vi "log analysis_gps.vi"() -> ()   [LabVIEW 2019] (continued)
-1.127697\t1.583662\t-32.920876\t0.305000\t0.018000\n\t\n15:22:00.9\tlog_raw\tgps_raw\t\tsystem status\tnormal 2 28.100000 0 0\trobot status\t261.941278\t86.398374\t9.062300\t-1.078955\t1.573300\t-32.941024\t0.301000\t0.007000\n\t\n15:22:01.4\tlog_raw\tgps_raw\t\tsystem status\tnormal 2 28.100000 0 0\trobot status\t262.053513\t86.309329\t9.068200\t-0.868450\t1.546924\t-32.927997\t0.298000\t0.007000\n\t\n15:22:02.0\tlog_raw\tgps_raw\t\tsystem status\tnormal 2 28.100000 0 0\trobot status\t262.166872\t86.221531\t9.074900\t-0.908194\t1.762279\t-32.906753\t0.245000\t0.087000\n\t\n15:22:02.4\tlog_raw\tgps_raw\t\tsystem status\tnormal 2 28.100000 0 0\trobot status\t262.277689\t86.134631\t9.082500\t-0.875214\t1.923337\t-32.852666\t0.299000\t0.013000\n\t\n15:22:02.9\tlog_raw\tgps_raw\t\tsystem status\tnormal 2 28.100000 0 0\trobot status\t262.391399\t86.045063\t9.089000\t-0.783137\t1.975369\t-32.776874\t0.269000\t0.061000\n\t\n15:22:03.5\tlog_raw\tgps_raw\t\tsystem status\tnormal 2 28.000000 0 0\trobot status\t262.504223\t85.954379\t9.093500\t-0.563717\t2.005742\t-32.598822\t0.285000\t0.030000\n\t\n15:22:04.0\tlog_raw\tgps_raw\t\tsystem status\tnormal 2 28.000000 0 0\trobot status\t262.618184\t85.864642\t9.098400\t-0.517536\t1.887240\t-32.402540\t0.248000\t0.088000\n\t\n15:22:04.5\tlog_raw\tgps_raw\t\tsystem status\tnormal 2 28.000000 0 0\trobot status\t262.731624\t85.777102\t9.103300\t-0.639169\t1.824657\t-32.135487\t0.298000\t0.023000\n\t\n15:22:05.0\tlog_raw\tgps_raw\t\tsystem status\tnormal 2 28.000000 0 0\trobot status\t262.844713\t85.688582\t9.107700\t-0.582082\t1.791841\t-31.777069\t0.254000\t0.086000\n\t\n15:22:05.5\tlog_raw\tgps_raw\t\tsystem status\tnormal 2 28.000000 0 0\trobot status\t262.958759\t85.600798\t9.111300\t-0.337992\t1.837116\t-31.424550\t0.285000\t0.033000\n\t\n15:22:06.0\tlog_raw\tgps_raw\t\tsystem status\tnormal 2 28.000000 0 0\trobot status\t263.072897\t85.514711\t9.115300\t-0.200500\t1.972169\t-31.081279\t0.354000\t-0.083000\n\t\n15:22:06.5\tlog_raw\tgps_raw\t\tsystem status\tnormal 2 28.000000 0 0\trobot status\t263.187931\t85.429939\t9.121600\t-0.367282\t2.009452\t-30.701830\t0.308000\t0.008000\n\t\n15:22:07.0\tlog_raw\tgps_raw\t\tsystem status\tnormal 2 28.000000 0 0\trobot status\t263.303633\t85.344679\t9.127600\t-0.513723\t1.945308\t-30.287535\t0.224000\t0.128000\n\t\n15:22:07.5\tlog_raw\tgps_raw\t\tsystem status\tnormal 2 28.000000 0 0\trobot status\t263.421743\t85.261380\t9.132600\t-0.628149\t2.007379\t-29.987443\t0.388000\t-0.102000\n\t\n15:22:08.0\tlog_raw\tgps_raw\t\tsystem status\tnormal 2 28.000000 0 0\trobot status\t263.537798\t85.177709\t9.137900\t-0.493038\t2.083654\t-29.751402\t0.249000\t0.095000\n\t\n15:22:08.5\tlog_raw\tgps_raw\t\tsystem status\tnormal 2 28.000000 0 0\trobot status\t263.656042\t85.092856\t9.141300\t-0.435654\t1.911480\t-29.579462\t0.215000\t0.132000\n\t\n15:22:09.0\tlog_raw\tgps_raw\t\tsystem status\tnormal 2 28.000000 0 0\trobot status\t263.775801\t85.009077\t9.144900\t-0.600511\t1.730684\t-29.385724\t0.415000\t-0.165000\n\t\n15:22:09.5\tlog_raw\tgps_raw\t\tsystem status\tnormal 2 28.000000 0 0\trobot status\t263.892502\t84.926945\t9.149700\t-0.589621\t1.751596\t-29.305777\t0.349000\t-0.083000\n\t\n15:22:10.0\tlog_raw\tgps_raw\t\tsystem status\tnormal 2 28.000000 0 0\trobot status\t264.010675\t84.845063\t9.154900\t-0.727270\t1.661816\t-29.246267\t0.279000\t0.023000\n\t\n15:22:10.5\tlog_raw\tgps_raw\t\tsystem status\tnormal 2 28.100000 0 0\trobot status\t264.130059\t84.763395\t9.160200\t-0.558660\t1.596900\t-29.181046\t0.306000\t-0.013000\n\t\n15:22:11.0\tlog_raw\tgps_raw\t\tsystem status\tnormal 2 28.100000 0 0\trobot status\t264.247679\t84.683991\t9.164600\t-0.545053\t1.607938\t-29.232310\t0.293000\t0.000000\n\t\n15:22:11.5\tlog_raw\tgps_raw\t\tsystem status\tnormal 2 28.100000 0 0\trobot status\t264.364964\t84.605638\t9.167900\t-0.657584\t1.566108\t-29.306229\t0.298000\t-0.005000\n\t\n15:22:12.0\tlog_raw\tgps_raw\t\tsystem status\tnormal 2 28.100000 0 0\trobot status\t264.482065\t84.525337\t9.171700\t-0.685140\t1.437536\t-29.325810\t0.299000\t-0.009000\n\t\n15:22:12.5\tlog_raw\tgps_raw\t\tsystem status\tnormal 2 28.100000 0 0\trobot status\t264.596622\t84.445756\t9.173900\t-0.636600\t1.591267\t-29.359965\t0.305000\t-0.005000\n\t\n15:22:13.0\tlog_raw\tgps_raw\t\tsystem status\tnormal 2 28.100000 0 0\trobot status\t264.712151\t84.364986\t9.176300\t-0.594728\t1.685918\t-29.442723\t0.299000\t-0.015000\n\t\n15:22:13.5\tlog_raw\tgps_raw\t#INSPVAXA,USB3,0,51.0,FINESTEERING,2107,282151.500,02000000,471d,15824;INS_ALIGNMENT_COMPLETE,INS_RTKFIXED,37.37088960505,126.72382499990,9.1778,22.3000,-0.1858,0.2425,0.0007,-0.584217482,1.708777597,119.499420224,0.4348,0.2933,0.5266,0.1137,0.0921,0.0762,0.1458,0.1498,5.0245,0f000001,0*a137cdab\n\tsystem status\tnormal 2 28.100000 0 0\trobot status\t264.839984\t84.278458\t9.177800\t-0.584217\t1.708778\t-29.499420\t0.302000\t-0.003000\n\t\n15:22:14.0\tlog_raw\tgps_raw\t\tsystem status\tnormal 2 28.100000 0 0\trobot status\t264.946789\t84.205330\t9.178700\t-0.520865\t1.632929\t-29.652181\t0.297000\t-0.013000\n\t\n15:22:14.5\tlog_raw\tgps_raw\t\tsystem status\tnormal 2 28.100000 0 0\trobot status\t265.065594\t84.123990\t9.181000\t-0.558139\t1.552308\t-29.875580\t0.296000\t-0.013000\n\t\n15:22:15.0\tlog_raw\tgps_raw\t\tsystem status\tnormal 2 28.100000 0 0\trobot status\t265.179580\t84.043869\t9.183300\t-0.583331\t1.445555\t-30.150948\t0.302000\t-0.015000\n\t\n15:22:15.5\tlog_raw\tgps_raw\t#INSPVAXA,USB3,0,46.5,FINESTEERING,2107,282153.500,02000000,471d,15824;INS_ALIGNMENT_COMPLETE,INS_RTKFIXED,37.37088668027,126.72383030308,9.1844,22.3000,-0.1846,0.2433,-0.0063,-0.490970731,1.271254139,120.414068071,0.4478,0.2935,0.5351,0.1145,0.0921,0.0767,0.1457,0.1497,5.0277,0f000001,0*2a0513c3\n\tsystem status\tnormal 2 28.100000 0 0\trobot status\t265.309731\t83.953838\t9.184400\t-0.490971\t1.271254\t-30.414068\t0.298000\t-0.019000\n\t\n15:22:16.0\tlog_raw\tgps_raw\t\tsystem status\tnormal 2 28.100000 0 0\trobot status\t265.417867\t83.878165\t9.184100\t-0.413269\t1.356131\t-30.605113\t0.300000\t-0.023000\n\t\n15:22:16.5\tlog_raw\tgps_raw\t#INSPVAXA,USB3,0,47.0,FINESTEERING,2107,282154.500,02000000,471d,15824;INS_ALIGNMENT_COMPLETE,INS_RTKFIXED,37.37088518540,126.72383296501,9.1848,22.3000,-0.1849,0.2389,0.0033,-0.578089293,1.343840193,120.921980586,0.4509,0.2935,0.5383,0.1145,0.0921,0.0767,0.1457,0.1497,5.0293,0f000001,0*6c2251c0\n\tsystem status\tnormal 2 28.100000 0 0\trobot status\t265.545521\t83.787923\t9.184800\t-0.578089\t1.343840\t-30.921981\t0.298000\t-0.014000\n\t\n15:22:17.0\tlog_raw\tgps_raw\t\tsystem status\tnormal 2 28.000000 0 0\trobot status\t265.649046\t83.712481\t9.185900\t-0.588736\t1.427335\t-31.143204\t0.298000\t-0.013000\n\t\n15:22:17.5\tlog_raw\tgps_raw\t\tsystem status\tnormal 2 28.100000 0 0\trobot status\t265.765763\t83.628763\t9.189700\t-0.499246\t1.474432\t-31.400120\t0.293000\t-0.005000\n\t\n15:22:18.0\tlog_raw\tgps_raw\t#INSPVAXA,USB3,0,49.5,FINESTEERING,2107,282156.000,02000000,471d,15824;INS_ALIGNMENT_COMPLETE,INS_RTKFIXED,37.37088292743,126.72383688922,9.1933,22.3000,-0.1804,0.2249,-0.0069,-0.526000833,1.617795510,121.650926042,0.4526,0.2935,0.5409,0.1144,0.0920,0.0768,0.1457,0.1496,5.0309,0f000001,0*7b06a300\n\tsystem status\tnormal 2 28.100000 0 0\trobot status\t265.893121\t83.537312\t9.193300\t-0.526001\t1.617796\t-31.650926\t0.293000\t-0.005000\n\t\n15:22:18.5\tlog_raw\tgps_raw\t#INSPVAXA,USB3,0,48.5,FINESTEERING,2107,282156.500,02000000,471d,15824;INS_ALIGNMENT_COMPLETE,INS_RTKFIXED,37.37088217363,126.72383817131,9.1964,22.3000,-0.1807,0.2394,-0.0085,-0.574321613,1.643212102,121.914347439,0.4534,0.2936,0.5427,0.1143,0.0921,0.0768,0.1456,0.1496,5.0325,0f000001,0*15ca3725\n\tsystem status\tnormal 2 28.100000 0 0\trobot status\t266.006686\t83.453648\t9.196400\t-0.574322\t1.643212\t-31.914347\t0.300000\t-0.011000\n\t\n15:22:19.0\tlog_raw\tgps_raw\t#INSPVAXA,USB3,0,48.5,FINESTEERING,2107,282157.000,02000000,471d,15824;INS_ALIGNMENT_COMPLETE,INS_RTKFIXED,37.37088140399,126.72383945930,9.1993,22.3000,-0.1862,0.2446,-0.0064,-0.600405217,1.496036608,122.180467270,0.4534,0.2936,0.5427,0.1143,0.0921,0.0768,0.1456,0.1496,5.0325,0f000001,0*c5e5c6e3\n\tsystem status\tnormal 2 28.100000 0 0\trobot status\t266.120774\t83.368226\t9.199300\t-0.600405\t1.496037\t-32.180467\t0.301000\t-0.007000\n\t\n15:22:19.5\tlog_raw\tgps_raw\t\tsystem status\tnormal 2 28.100000 0 0\trobot status\t266.223466\t83.290507\t9.201700\t-0.489393\t1.491418\t-32.380033\t0.300000\t-0.003000\n\t\n15:22:20.0\tlog_raw\tgps_raw\t\tsystem status\tnormal 2 28.100000 0 0\trobot status\t266.335395\t83.205661\t9.205500\t-0.537253\t1.491739\t-32.667666\t0.300000\t-0.008000\n\t\n15:22:20.5\tlog_raw\tgps_raw\t#INSPVAXA,USB3,0,45.5,FINESTEERING,2107,282158.500,02000000,471d,15824;INS_ALIGNMENT_COMPLETE,INS_RTKFIXED,37.37087907876,126.72384326761,9.2104,22.3000,-0.1767,0.2291,0.0108,-0.395230088,1.351210238,122.917750135,0.4537,0.2937,0.5451,0.1144,0.0921,0.0768,0.1456,0.1495,5.0357,0f000001,0*07daf6c2\n\tsystem status\tnormal 2 28.100000 0 0\trobot status\t266.458108\t83.110151\t9.210400\t-0.395230\t1.351210\t-32.917750\t0.300000\t0.000000\n\t\n15:22:21.0\tlog_raw\tgps_raw\t#INSPVAXA,USB3,0,45.5,FINESTEERING,2107,282159.000,02000000,471d,15824;INS_ALIGNMENT_COMPLETE,INS_RTKFIXED,37.37087827658,126.72384453527,9.2150,22.3000,-0.1825,0.2336,0.0127,-0.281125763,1.400376320,123.162742277,0.4537,0.2937,0.5451,0.1144,0.0921,0.0768,0.1456,0.1495,5.0357,0f000001,0*5700aa0a\n\tsystem status\tnormal 2 28.100000 0 0\trobot status\t266.570395\t83.021117\t9.215000\t-0.281126\t1.400376\t-33.162742\t0.301000\t0.000000\n\t\n15:22:21.5\tlog_raw\tgps_raw\t\tsystem status\tnormal 2 28.100000 0 0\trobot status\t266.671836\t82.944090\t9.218400\t-0.235676\t1.388791\t-33.352805\t0.302000\t0.005000\n\t\n15:22:22.0\tlog_raw\tgps_raw\t\tsystem status\tnormal 2 28.100000 0 0\trobot status\t266.783087\t82.858226\t9.223700\t-0.198184\t1.436943\t-33.469917\t0.302000\t0.003000\n\t\n15:22:22.5\tlog_raw\tgps_raw\t\tsystem status\tnormal 2 28.100000 0 0\trobot status\t266.897329\t82.770367\t9.230100\t-0.166769\t1.482305\t-33.474248\t0.298000\t0.015000\n\t\n15:22:23.0\tlog_raw\tgps_raw\t#INSPVAXA,USB3,0,48.5,FINESTEERING,2107,282161.000,02000000,471d,15824;INS_ALIGNMENT_COMPLETE,INS_RTKFIXED,37.37087514986,126.72384964420,9.2386,22.3000,-0.1845,0.2318,0.0206,-0.134311793,1.526790970,123.449672080,0.4533,0.2938,0.5460,0.1147,0.0921,0.0768,0.1455,0.1496,5.0387,0f000001,0*1e397fdc\n\tsystem status\tnormal 2 28.100000 0 0\trobot status\t267.022936\t82.674085\t9.238600\t-0.134312\t1.526791\t-33.449672\t0.300000\t0.016000\n\t\n15:22:23.5\tlog_raw\tgps_raw\t\tsystem status\tnormal 2 28.100000 0 0\trobot status\t267.126884\t82.594063\t9.244300\t-0.120862\t1.476797\t-33.495215\t0.300000\t0.007000\n\t\n15:22:24.0\tlog_raw\tgps_raw\t#INSPVAXA,USB3,0,49.0,FINESTEERING,2107,282162.000,02000000,471d,15824;INS_ALIGNMENT_COMPLETE,INS_RTKFIXED,37.37087356615,126.72385221886,9.2529,22.3000,-0.1851,0.2394,-0.0036,-0.080021339,1.630723538,123.455447603,0.4532,0.2939,0.5462,0.1148,0.0921,0.0768,0.1454,0.1496,5.0402,0f000001,0*5854c212\n\tsystem status\tnormal 2 28.100000 0 0\trobot status\t267.250995\t82.498311\t9.252900\t-0.080021\t1.630724\t-33.455448\t0.304000\t0.006000\n\t\n15:22:24.5\tlog_raw\tgps_raw\t#INSPVAXA,USB3,0,51.0,FINESTEERING,2107,282162.500,02000000,471d,15824;INS_ALIGNMENT_COMPLETE,INS_RTKFIXED,37.37087276598,126.72385350535,9.2616,22.3000,-0.1911,0.2293,0.0115,-0.073182754,1.698964868,123.450820933,0.4532,0.2939,0.5462,0.1150,0.0921,0.0768,0.1454,0.1496,5.0417,0f000001,0*35a5fbef\n\tsystem status\tnormal 2 28.100000 0 0\trobot status\t267.364950\t82.409500\t9.261600\t-0.073183\t1.698965\t-33.450821\t0.293000\t0.016000\n\t\n15:22:25.0\tlog_raw\tgps_raw\t#INSPVAXA,USB3,0,51.0,FINESTEERING,2107,282163.000,02000000,471d,15824;INS_ALIGNMENT_COMPLETE,INS_RTKFIXED,37.37087198418,126.72385476769,9.2713,22.3000,-0.1886,0.2265,0.0207,-0.163897307,1.756288597,123.387194402,0.4532,0.2939,0.5462,0.1150,0.0921,0.0768,0.1454,0.1496,5.0417,0f000001,0*f7296fb4\n\tsystem status\tnormal 2 28.000000 0 0\trobot status\t267.476766\t82.322729\t9.271300\t-0.163897\t1.756289\t-33.387194\t0.349000\t-0.070000\n\t\n15:22:25.5\tlog_raw\tgps_raw\t#INSPVAXA,USB3,0,50.0,FINESTEERING,2107,282163.500,02000000,471d,15824;INS_ALIGNMENT_COMPLETE,INS_RTKFIXED,37.37087116734,126.72385603736,9.2795,22.3000,-0.1822,0.2264,0.0180,-0.228587283,1.950230328,123.198406451,0.4532,0.2939,0.5462,0.1150,0.0921,0.0768,0.1454,0.1496,5.0417,0f000001,0*1ae1e07b\n\tsystem status\tnormal 2 28.000000 0 0\trobot status\t267.589232\t82.232069\t9.279500\t-0.228587\t1.950230\t-33.198406\t0.251000\t0.076000\n\t\n15:22:26.0\tlog_raw\tgps_raw\t#INSPVAXA,USB3,0,50.0,FINESTEERING,2107,282164.000,02000000,471d,15824;INS_ALIGNMENT_COMPLETE,INS_RTKFIXED,37.37087034978,126.72385731621,9.2879,22.3000,-0.1896,0.2295,0.0123,-0.289631727,1.840561194,122.888440752,0.4532,0.2939,0.5462,0.1150,0.0921,0.0768,0.1454,0.1496,5.0417,0f000001,0*056b33eb\n\tsystem status\tnormal 2 28.000000 0 0\trobot status\t267.702510\t82.141329\t9.287900\t-0.289632\t1.840561\t-32.888441\t0.322000\t-0.019000\n\t\n15:22:26.5\tlog_raw\tgps_raw\t#INSPVAXA,USB3,0,49.5,FINESTEERING,2107,282164.500,02008000,471d,15824;INS_ALIGNMENT_COMPLETE,INS_RTKFIXED,37.37086961397,126.72385855899,9.2957,22.3000,-0.1725,0.2178,0.0037,-0.245083318,1.835832496,122.519490120,0.5068,0.3317,0.5928,0.1224,0.0977,0.0793,0.1462,0.1507,5.0448,0f000001,0*242e4928\n\tsystem status\tnormal 2 28.000000 0 0\trobot status\t267.812594\t82.059661\t9.295700\t-0.245083\t1.835832\t-32.519490\t0.311000\t-0.006000\n\t\n15:22:27.0\tlog_raw\tgps_raw\t#INSPVAXA,USB3,0,49.5,FINESTEERING,2107,282165.000,02008000,471d,15824;INS_ALIGNMENT_COMPLETE,INS_RTKFIXED,37.37086887660,126.72385979146,9.3053,22.3000,-0.1797,0.2392,0.0086,-0.083873160,1.728047221,122.128251979,0.5068,0.3317,0.5928,0.1224,0.0977,0.0793,0.1462,0.1507,5.0448,0f000001,0*7f8693c0\n\tsystem status\tnormal 2 28.000000 0 0\trobot status\t267.921764\t81.977821\t9.305300\t-0.083873\t1.728047\t-32.128252\t0.404000\t-0.145000\n\t\n15:22:27.5\tlog_raw\tgps_raw\t#INSPVAXA,USB3,0,50.0,FINESTEERING,2107,282165.500,02008000,471d,15824;INS_ALIGNMENT_COMPLETE,INS_RTKFIXED,37.37086811316,126.72386104230,9.3143,22.3000,-0.1621,0.2209,0.0106,0.024861587,1.649578148,121.656445407,0.4863,0.3145,0.5830,0.1190,0.0946,0.0782,0.1458,0.1502,5.0461,0f000001,0*34f23d42\n\tsystem status\tnormal 2 27.900000 0 0\trobot status\t268.032561\t81.893088\t9.314300\t0.024862\t1.649578\t-31.656445\t0.277000\t0.036000\n\t\n15:22:28.0\tlog_raw\tgps_raw\t#INSPVAXA,USB3,0,50.0,FINESTEERING,2107,282166.000,02008000,471d,15824;INS_ALIGNMENT_COMPLETE,INS_RTKFIXED,37.37086751829,126.72386195729,9.3219,22.3000,-0.0093,-0.0451,0.0007,-0.021903893,1.492441336,121.617580212,0.4863,0.3145,0.5830,0.1190,0.0946,0.0782,0.1458,0.1502,5.0461,0f000001,0*e5b24ae3\n\tsystem status\tnormal 2 28.000000 0 0\trobot status\t268.113609\t81.827064\t9.321900\t-0.021904\t1.492441\t-31.617580\t0.074000\t-0.199000\n\t\n15:22:28.5\tlog_raw\tgps_raw\t#INSPVAXA,USB3,0,48.5,FINESTEERING,2107,282166.500,02008000,471d,15824;INS_ALIGNMENT_COMPLETE,INS_RTKFIXED,37.37086745954,126.72386181526,9.3232,22.3000,-0.0268,-0.0236,0.0089,-0.043372783,1.566427448,121.563343894,0.4732,0.3047,0.5748,0.1189,0.0947,0.0774,0.1456,0.1500,5.0475,0f000001,0*3570ed60\n\tsystem status\tnormal 2 28.100000 0 0\trobot status\t268.101029\t81.820544\t9.323200\t-0.043373\t1.566427\t-31.563344\t-0.001000\t0.000000\n\t\n15:22:29.0\tlog_raw\tgps_raw\t#INSPVAXA,USB3,0,48.5,FINESTEERING,2107,282167.000,02008000,471d,15824;INS_ALIGNMENT_COMPLETE,INS_RTKFIXED,37.37086722262,126.72386202898,9.3264,22.3000,-0.1700,0.2085,0.0159,-0.059764704,1.681922525,121.297414016,0.4732,0.3047,0.5748,0.1189,0.0947,0.0774,0.1456,0.1500,5.0475,0f000001,0*686f29fa\n\tsystem status\tnormal 2 28.000000 0 0\trobot status\t268.119960\t81.794249\t9.326400\t-0.059765\t1.681923\t-31.297414\t0.269000\t0.004000\n\t\n15:22:29.5\tlog_raw\tgps_raw\t#INSPVAXA,USB3,0,51.0,FINESTEERING,2107,282167.500,02008000,471d,15824;INS_ALIGNMENT_COMPLETE,INS_RTKFIXED,37.37086635075,126.72386343693,9.3355,22.3000,-0.1343,0.1551,0.0138,-0.191041256,1.725233794,121.448181107,0.4732,0.3047,0.5748,0.1189,0.0947,0.0774,0.1456,0.1500,5.0475,0f000001,0*c09661b1\n\tsystem status\tnormal 2 28.100000 0 0\trobot status\t268.244673\t81.697480\t9.335500\t-0.191041\t1.725234\t-31.448181\t0.195000\t0.099000\n\t\n15:22:30.0\tlog_raw\tgps_raw\t#INSPVAXA,USB3,0,51.0,FINESTEERING,2107,282168.000,02008000,471d,15824;INS_ALIGNMENT_COMPLETE,INS_RTKFIXED,37.37086554629,126.72386469627,9.3449,22.3000,-0.1443,0.1947,0.0175,-0.193885511,1.717406727,121.172307594,0.4732,0.3047,0.5748,0.1189,0.0947,0.0774,0.1456,0.1500,5.0475,0f000001,0*05ac97bf\n\tsystem status\tnormal 2 28.000000 0 0\trobot status\t268.356224\t81.608194\t9.344900\t-0.193886\t1.717407\t-31.172308\t0.374000\t-0.085000\n\t\n15:22:30.5\tlog_raw\tgps_raw\t#INSPVAXA,USB3,0,51.0,FINESTEERING,2107,282168.500,02000000,471d,15824;INS_ALIGNMENT_COMPLETE,INS_RTKFIXED,37.37086484906,126.72386602613,9.3508,22.3000,-0.1684,0.2118,0.0292,-0.052015142,1.767687292,120.756942814,0.5200,0.3367,0.6136,0.1257,0.1009,0.0794,0.1465,0.1509,5.0427,0f000001,0*74b10fb1\n\tsystem status\tnormal 2 28.000000 0 0\trobot status\t268.474021\t81.530809\t9.350800\t-0.052015\t1.767687\t-30.756943\t0.336000\t-0.029000\n\t\n15:22:31.0\tlog_raw\tgps_raw\t#INSPVAXA,USB3,0,51.0,FINESTEERING,2107,282169.000,02000000,471d,15824;INS_ALIGNMENT_COMPLETE,INS_RTKFIXED,37.37086415822,126.72386736868,9.3575,22.3000,-0.1707,0.2211,0.0151,0.018670150,1.718273405,120.397652354,0.5200,0.3367,0.6136,0.1257,0.1009,0.0794,0.1465,0.1509,5.0427,0f000001,0*7f0a75ca\n\tsystem status\tnormal 2 28.000000 0 0\trobot status\t268.592941\t81.454132\t9.357500\t0.018670\t1.718273\t-30.397652\t0.279000\t0.047000\n\t\n15:22:31.5\tlog_raw\tgps_raw\t#INSPVAXA,USB3,0,46.0,FINESTEERING,2107,282169.500,02000000,471d,15824;INS_ALIGNMENT_COMPLETE,INS_RTKFIXED,37.37086344397,126.72386871844,9.3630,22.3000,-0.1742,0.2275,0.0011,-0.016191041,1.633927809,119.983496476,0.4955,0.3175,0.5974,0.1215,0.0969,0.0780,0.1460,0.1504,5.0326,0f000001,0*70440743\n\tsystem status\tnormal 2 28.000000 0 0\trobot status\t268.712501\t81.374858\t9.363000\t-0.016191\t1.633928\t-29.983496\t0.245000\t0.074000\n\t\n15:22:32.0\tlog_raw\tgps_raw\t#DUALANTENNAHEADINGA,USB3,0,46.0,FINESTEERING,2107,282170.000,02000000,d426,15824;INSUFFICIENT_OBS,NONE,0.000000000,0.000000000,0.000000000,0.0,0.000000000,0.000000000,\"\",0,0,0,0,00,00,00,00*d9bd9ff7\n\tsystem status\tnormal 2 28.000000 0 0\trobot status\t268.830910\t81.295954\t9.369000\t-0.045104\t1.608513\t-29.594999\t0.282000\t0.035000\n\t\n15:22:32.5\tlog_raw\tgps_raw\t#INSPVAXA,USB3,0,49.5,FINESTEERING,2107,282170.500,02000000,471d,15824;INS_ALIGNMENT_COMPLETE,INS_RTKFIXED,37.37086196149,126.72387133593,9.3775,22.3000,-0.1638,0.2319,0.0101,-0.134678922,1.597363801,119.344832889,0.4955,0.3175,0.5974,0.1215,0.0969,0.0780,0.1460,0.1504,5.0326,0f000001,0*0ad13adf\n\tsystem status\tnormal 2 28.000000 0 0\trobot status\t268.944354\t81.210318\t9.377500\t-0.134679\t1.597364\t-29.344833\t0.354000\t-0.086000\n\t\n15:22:33.0\tlog_raw\tgps_raw\t#INSPVAXA,USB3,0,49.5,FINESTEERING,2107,282171.000,02000000,471d,15824;INS_ALIGNMENT_COMPLETE,INS_RTKFIXED,37.37086118756,126.72387260380,9.3866,22.3000,-0.1780,0.2223,0.0226,-0.237576400,1.617402983,119.136823599,0.4955,0.3175,0.5974,0.1215,0.0969,0.0780,0.1460,0.1504,5.0326,0f000001,0*d3c2583e\n\tsystem status\tnormal 2 28.000000 0 0\trobot status\t269.056660\t81.124420\t9.386600\t-0.237576\t1.617403\t-29.136824\t0.283000\t0.016000\n\t\n15:22:33.5\tlog_raw\tgps_raw\t#DUALANTENNAHEADINGA,USB3,0,52.5,FINESTEERING,2107,282171.500,02000000,d426,15824;SOL_COMPUTED,L1_FLOAT,-1.000000000,212.575851440,56.383117676,0.0,44.713680267,134.992919922,\"631T\",11,5,5,5,04,00,20,02*bb8370c9\n\tsystem status\tnormal 2 28.000000 0 0\trobot status\t269.168042\t81.037548\t9.396200\t-0.254862\t1.734252\t-28.972869\t0.311000\t-0.011000\n\t\n15:22:34.0\tlog_raw\tgps_raw\t#INSPVAXA,USB3,0,52.5,FINESTEERING,2107,282172.000,02000000,471d,15824;INS_ALIGNMENT_COMPLETE,INS_RTKFIXED,37.37085961658,126.72387509904,9.4055,22.3000,-0.1866,0.2197,0.0120,-0.164173617,1.908755927,118.881251858,0.4955,0.3175,0.5974,0.1215,0.0969,0.0780,0.1460,0.1504,5.0326,0f000001,0*7b1cb490\n\tsystem status\tnormal 2 28.000000 0 0\trobot status\t269.277684\t80.950058\t9.405500\t-0.164174\t1.908756\t-28.881252\t0.339000\t-0.049000\n\t\n15:22:34.5\tlog_raw\tgps_raw\t#DUALANTENNAHEADINGA,USB3,0,51.0,FINESTEERING,2107,282172.500,02008000,d426,15824;SOL_COMPUTED,NARROW_FLOAT,-1.000000000,128.001327515,-71.010498047,0.0,360.000000000,151.438781738,\"631T\",13,7,7,5,04,00,20,03*76c36059\n\tsystem status\tnormal 2 28.000000 0 0\trobot status\t269.403666\t80.879283\t9.406100\t-0.214673\t1.991228\t-28.883399\t0.281000\t0.013000\n\t\n15:22:35.0\tlog_raw\tgps_raw\t#INSPVAXA,USB3,0,51.0,FINESTEERING,2107,282173.000,02008000,471d,15824;INS_ALIGNMENT_COMPLETE,INS_RTKFIXED,37.37085833527,126.72387797741,9.4066,22.3000,-0.1810,0.2279,0.0198,-0.406869052,2.030704243,118.923772886,0.5770,0.3723,0.6754,0.1336,0.1058,0.0814,0.1476,0.1521,5.0145,0f000001,0*4f67786d\n\tsystem status\tnormal 2 28.100000 0 0\trobot status\t269.532645\t80.807844\t9.406600\t-0.406869\t2.030704\t-28.923773\t0.303000\t-0.006000\n\t\n15:22:35.5\tlog_raw\tgps_raw\t#INSPVAXA,USB3,0,51.0,FINESTEERING,2107,282173.500,02008000,471d,15824;INS_ALIGNMENT_COMPLETE,INS_RTKFIXED,37.37085763620,126.72387935658,9.4103,22.3000,-0.1736,0.2330,0.0207,-0.517446305,1.873578132,118.931812586,0.5249,0.3329,0.6407,0.1266,0.1009,0.0786,0.1470,0.1512,5.0071,0f000001,0*4ebf01a6\n\tsystem status\tnormal 2 28.000000 0 0\trobot status\t269.654810\t80.730254\t9.410300\t-0.517446\t1.873578\t-28.931813\t0.299000\t-0.002000\n\t\n15:22:36.0\tlog_raw\tgps_raw\t#DUALANTENNAHEADINGA,USB3,0,51.0,FINESTEERING,2107,282174.000,02008000,d426,15824;SOL_COMPUTED,NARROW_FLOAT,-1.000000000,123.069808960,-65.629364014,0.0,360.000000000,180.000000000,\"631T\",16,6,6,5,04,00,20,03*92b169c2\n\tsystem status\tnormal 2 28.100000 0 0\trobot status\t269.777456\t80.650245\t9.413500\t-0.518049\t1.628021\t-28.970226\t0.296000\t-0.008000\n\t\n15:22:36.5\tlog_raw\tgps_raw\t#DUALANTENNAHEADINGA,USB3,0,49.0,FINESTEERING,2107,282174.500,02008000,d426,15824;SOL_COMPUTED,NARROW_FLOAT,-1.000000000,124.551315308,-68.632659912,0.0,360.000000000,180.000000000,\"631T\",16,7,7,5,04,00,20,03*6a9e420e\n\tsystem status\tnormal 2 28.100000 0 0\trobot status\t269.895249\t80.570496\t9.417300\t-0.440481\t1.445201\t-29.004640\t0.302000\t-0.010000\n\t\n15:22:37.0\tlog_raw\tgps_raw\t#INSPVAXA,USB3,0,49.0,FINESTEERING,2107,282175.000,02008000,471d,15824;INS_ALIGNMENT_COMPLETE,INS_RTKFIXED,37.37085549477,126.72388337891,9.4209,22.3000,-0.1860,0.2237,0.0201,-0.564638995,1.417085276,119.025707092,0.4961,0.3139,0.6151,0.1240,0.1000,0.0771,0.1467,0.1509,5.0036,0f000001,0*2746038f\n\tsystem status\tnormal 2 28.100000 0 0\trobot status\t270.011101\t80.492577\t9.420900\t-0.564639\t1.417085\t-29.025707\t0.304000\t-0.015000\n\t\n15:22:37.5\tlog_raw\tgps_raw\t#INSPVAXA,USB3,0,50.0,FINESTEERING,2107,282175.500,02008000,471d,15824;INS_ALIGNMENT_COMPLETE,INS_RTKFIXED,37.37085479315,126.72388469742,9.4248,22.3000,-0.1822,0.2271,0.0141,-0.513806522,1.414717204,119.104354508,0.4791,0.3046,0.5957,0.1234,0.0999,0.0764,0.1464,0.1507,5.0029,0f000001,0*e3204e40\n\tsystem status\tnormal 2 28.100000 0 0\trobot status\t270.127893\t80.414704\t9.424800\t-0.513807\t1.414717\t-29.104355\t0.301000\t-0.006000\n\t\n15:22:38.0\tlog_raw\tgps_raw\t#INSPVAXA,USB3,0,50.0,FINESTEERING,2107,282176.000,02008000,471d,15824;INS_ALIGNMENT_COMPLETE,INS_RTKFIXED,37.37085410326,126.72388599341,9.4283,22.3000,-0.1760,0.2106,0.0151,-0.605541417,1.454743259,119.281713752,0.4791,0.3046,0.5957,0.1234,0.0999,0.0764,0.1464,0.1507,5.0029,0f000001,0*bcb93fc8\n\tsystem status\tnormal 2 28.100000 0 0\trobot status\t270.242690\t80.338133\t9.428300\t-0.605541\t1.454743\t-29.281714\t0.299000\t-0.015000\n\t\n15:22:38.5\tlog_raw\tgps_raw\t#DUALANTENNAHEADINGA,USB3,0,48.5,FINESTEERING,2107,282176.500,02000000,d426,15824;SOL_COMPUTED,NARROW_FLOAT,-1.000000000,134.305130005,-57.419616699,0.0,360.000000000,180.000000000,\"631T\",18,6,6,5,04,00,20,03*ffb18b5f\n\tsystem status\tnormal 2 28.100000 0 0\trobot status\t270.360254\t80.258468\t9.432900\t-0.628661\t1.506658\t-29.477693\t0.295000\t-0.017000\n\t\n15:22:39.0\tlog_raw\tgps_raw\t#DUALANTENNAHEADINGA,USB3,0,48.5,FINESTEERING,2107,282177.000,02000000,d426,15824;SOL_COMPUTED,NARROW_FLOAT,-1.000000000,135.311111450,-57.297637939,0.0,360.000000000,180.000000000,\"631T\",18,6,6,5,04,00,20,03*ffb49dec\n\tsystem status\tnormal 2 28.100000 0 0\trobot status\t270.476900\t80.177583\t9.438300\t-0.591807\t1.534856\t-29.752462\t0.299000\t-0.020000\n\t\n15:22:39.5\tlog_raw\tgps_raw\t#INSPVAXA,USB3,0,48.0,FINESTEERING,2107,282177.500,02000000,471d,15824;INS_ALIGNMENT_COMPLETE,INS_RTKFIXED,37.37085188860,126.72389002075,9.4437,22.3000,-0.1883,0.2420,0.0164,-0.505003517,1.427423679,120.083460934,0.4645,0.2990,0.5702,0.1231,0.0988,0.0761,0.1455,0.1502,5.0044,0f000001,0*390fa34e\n\tsystem status\tnormal 2 28.100000 0 0\trobot status\t270.599425\t80.092328\t9.443700\t-0.505004\t1.427424\t-30.083461\t0.301000\t-0.024000\n\t\n15:22:40.0\tlog_raw\tgps_raw\t#INSPVAXA,USB3,0,48.0,FINESTEERING,2107,282178.000,02000000,471d,15824;INS_ALIGNMENT_COMPLETE,INS_RTKFIXED,37.37085112539,126.72389137243,9.4485,22.3000,-0.1737,0.2237,0.0239,-0.447467240,1.418285202,120.360306359,0.4645,0.2990,0.5702,0.1231,0.0988,0.0761,0.1455,0.1502,5.0044,0f000001,0*ee66b8d3\n\tsystem status\tnormal 2 28.100000 0 0\trobot status\t270.719154\t80.007620\t9.448500\t-0.447467\t1.418285\t-30.360306\t0.298000\t-0.023000\n\t\n15:22:40.5\tlog_raw\tgps_raw\t#DUALANTENNAHEADINGA,USB3,0,48.5,FINESTEERING,2107,282178.500,02000000,d426,15824;SOL_COMPUTED,L1_FLOAT,-1.000000000,214.039077759,54.311355591,0.0,31.311414719,120.360610962,\"631T\",17,5,5,5,04,00,20,02*7f9a84dc\n\tsystem status\tnormal 2 28.100000 0 0\trobot status\t270.837205\t79.925754\t9.453100\t-0.698470\t1.564491\t-30.635562\t0.305000\t-0.016000\n\t\n15:22:41.0\tlog_raw\tgps_raw\t#INSPVAXA,USB3,0,48.5,FINESTEERING,2107,282179.000,02000000,471d,15824;INS_ALIGNMENT_COMPLETE,INS_RTKFIXED,37.37084962670,126.72389402617,9.4575,22.3000,-0.1964,0.2240,0.0138,-0.716798061,1.635103136,120.928637388,0.4619,0.2984,0.5621,0.1226,0.0976,0.0763,0.1451,0.1499,5.0052,0f000001,0*33d16cf5\n\tsystem status\tnormal 2 28.000000 0 0\trobot status\t270.954218\t79.841281\t9.457500\t-0.716798\t1.635103\t-30.928637\t0.312000\t-0.005000\n\t\n15:22:41.5\tlog_raw\tgps_raw\t#INSPVAXA,USB3,0,50.0,FINESTEERING,2107,282179.500,02000000,471d,15824;INS_ALIGNMENT_COMPLETE,INS_RTKFIXED,37.37084886052,126.72389534484,9.4614,22.3000,-0.1928,0.2247,0.0047,-0.502133863,1.643703431,121.221936688,0.4606,0.2980,0.5561,0.1219,0.0962,0.0765,0.1448,0.1496,5.0057,0f000001,0*d5b8afd0\n\tsystem status\tnormal 2 28.100000 0 0\trobot status\t271.071024\t79.756243\t9.461400\t-0.502134\t1.643703\t-31.221937\t0.312000\t-0.010000\n\t\n15:22:42.0\tlog_raw\tgps_raw\t#INSPVAXA,USB3,0,50.0,FINESTEERING,2107,282180.000,02000000,471d,15824;INS_ALIGNMENT_COMPLETE,INS_RTKFIXED,37.37084808459,126.72389666090,9.4649,22.3000,-0.1925,0.2192,0.0119,-0.378680064,1.659778733,121.498244377,0.4606,0.2980,0.5561,0.1219,0.0962,0.0765,0.1448,0.1496,5.0057,0f000001,0*ef9263b5\n\tsystem status\tnormal 2 28.100000 0 0\trobot status\t271.187598\t79.670123\t9.464900\t-0.378680\t1.659779\t-31.498244\t0.301000\t-0.019000\n\t\n15:22:42.5\tlog_raw\tgps_raw\t#DUALANTENNAHEADINGA,USB3,0,50.0,FINESTEERING,2107,282180.500,02000000,d426,15824;INSUFFICIENT_OBS,NONE,0.000000000,0.000000000,0.000000000,0.0,0.000000000,0.000000000,\"\",0,0,0,0,00,00,00,00*7c3513f7\n\tsystem status\tnormal 2 28.100000 0 0\trobot status\t271.298382\t79.578220\t9.473700\t-0.464234\t1.674060\t-31.849571\t0.304000\t-0.013000\n\t\n15:22:43.0\tlog_raw\tgps_raw\t#DUALANTENNAHEADINGA,USB3,0,50.0,FINESTEERING,2107,282181.000,02000000,d426,15824;INSUFFICIENT_OBS,NONE,0.000000000,0.000000000,0.000000000,0.0,0.000000000,0.000000000,\"\",0,0,0,0,00,00,00,00*d5a670f0\n\tsystem status\tnormal 2 28.100000 0 0\trobot status\t271.411819\t79.482048\t9.482000\t-0.592879\t1.514682\t-32.174211\t0.301000\t-0.006000\n\t\n15:22:43.5\tlog_raw\tgps_raw\t#DUALANTENNAHEADINGA,USB3,0,51.0,FINESTEERING,2107,282181.500,02000000,d426,15824;SOL_COMPUTED,L1_FLOAT,-1.000000000,135.320739746,-67.288024902,0.0,360.000000000,180.000000000,\"631T\",16,6,6,4,04,00,20,03*b9d4ea0f\n\tsystem status\tnormal 2 28.000000 0 0\trobot status\t271.519489\t79.385271\t9.489600\t-0.486070\t1.437066\t-32.469164\t0.300000\t-0.003000\n\t\n15:22:44.0\tlog_raw\tgps_raw\t#DUALANTENNAHEADINGA,USB3,0,51.0,FINESTEERING,2107,282182.000,02000000,d426,15824;SOL_COMPUTED,L1_FLOAT,-1.000000000,135.798538208,-66.526153564,0.0,360.000000000,180.000000000,\"631T\",19,6,6,3,04,00,20,00*2967dc6a\n\tsystem status\tnormal 2 28.100000 0 0\trobot status\t271.626468\t79.287903\t9.497100\t-0.531421\t1.310970\t-32.719245\t0.294000\t-0.003000\n\t\n15:22:44.5\tlog_raw\tgps_raw\t#INSPVAXA,USB3,0,49.0,FINESTEERING,2107,282182.500,02000000,471d,15824;INS_ALIGNMENT_COMPLETE,INS_RTKFIXED,37.37084393721,126.72390297520,9.4968,22.3000,-0.2002,0.2134,0.0137,-0.651107521,1.170361863,122.939925996,0.5624,0.3670,0.6434,0.1330,0.1041,0.0813,0.1464,0.1511,5.0059,0f000001,0*617b26b7\n\tsystem status\tnormal 2 28.100000 0 0\trobot status\t271.746909\t79.209809\t9.496800\t-0.651108\t1.170362\t-32.939926\t0.294000\t0.006000\n\t\n15:22:45.0\tlog_raw\tgps_raw\t#DUALANTENNAHEADINGA,USB3,0,49.0,FINESTEERING,2107,282183.000,02000000,d426,15824;INSUFFICIENT_OBS,NONE,0.000000000,0.000000000,0.000000000,0.0,0.000000000,0.000000000,\"\",0,0,0,0,00,00,00,00*b274769d\n\tsystem status\tnormal 2 28.100000 0 0\trobot status\t271.863769\t79.132378\t9.496200\t-0.646304\t1.083764\t-33.140847\t0.295000\t0.019000\n\t\n15:22:45.5\tlog_raw\tgps_raw\t#DUALANTENNAHEADINGA,USB3,0,47.0,FINESTEERING,2107,282183.500,02000000,d426,15824;INSUFFICIENT_OBS,NONE,0.000000000,0.000000000,0.000000000,0.0,0.000000000,0.000000000,\"\",0,0,0,0,00,00,00,00*9278fa5b\n\tsystem status\tnormal 2 28.100000 0 0\trobot status\t271.966072\t79.037100\t9.503200\t-0.572750\t1.159472\t-33.338852\t0.296000\t0.007000\n\t\n15:22:46.0\tlog_raw\tgps_raw\t#DUALANTENNAHEADINGA,USB3,0,47.0,FINESTEERING,2107,282184.000,02000000,d426,15824;INSUFFICIENT_OBS,NONE,0.000000000,0.000000000,0.000000000,0.0,0.000000000,0.000000000,\"\",0,0,0,0,00,00,00,00*4a16a1eb\n\tsystem status\tnormal 2 28.100000 0 0\trobot status\t272.072214\t78.936673\t9.510200\t-0.446247\t1.252374\t-33.416133\t0.298000\t0.006000\n\t\n15:22:46.5\tlog_raw\tgps_raw\t#DUALANTENNAHEADINGA,USB3,0,49.0,FINESTEERING,2107,282184.500,02000000,d426,15824;SOL_COMPUTED,NARROW_FLOAT,-1.000000000,146.879547119,-70.479187012,0.0,360.000000000,121.135261536,\"631T\",18,7,7,5,04,00,20,03*9a26e641\n\tsystem status\tnormal 2 28.100000 0 0\trobot status\t272.182740\t78.832728\t9.517300\t-0.504378\t1.261691\t-33.512666\t0.296000\t0.012000\n\t\n15:22:47.0\tlog_raw\tgps_raw\t#DUALANTENNAHEADINGA,USB3,0,49.0,FINESTEERING,2107,282185.000,02000000,d426,15824;SOL_COMPUTED,NARROW_FLOAT,-1.000000000,146.221954346,-70.420104980,0.0,360.000000000,123.181526184,\"631T\",18,7,7,5,04,00,20,03*8e5bbb52\n\tsystem status\tnormal 2 28.100000 0 0\trobot status\t272.293155\t78.727528\t9.524200\t-0.542538\t1.150373\t-33.551536\t0.299000\t0.014000\n\t\n15:22:47.5\tlog_raw\tgps_raw\t#DUALANTENNAHEADINGA,USB3,0,46.5,FINESTEERING,2107,282185.500,02000000,d426,15824;INSUFFICIENT_OBS,NONE,0.000000000,0.000000000,0.000000000,0.0,0.000000000,0.000000000,\"\",0,0,0,0,00,00,00,00*a89f4c07\n\tsystem status\tnormal 2 28.100000 0 0\trobot status\t272.421256\t78.655814\t9.522600\t-0.465015\t1.106299\t-33.462432\t0.297000\t0.016000\n\t\n15:22:48.0\tlog_raw\tgps_raw\t#INSPVAXA,USB3,0,46.5,FINESTEERING,2107,282186.000,02000000,471d,15824;INS_ALIGNMENT_COMPLETE,INS_RTKFIXED,37.37083829479,126.72391206471,9.5210,22.3000,-0.2075,0.2040,0.0190,-0.387614347,1.152152032,123.294354417,0.6060,0.3885,0.7100,0.1370,0.1076,0.0827,0.1473,0.1517,5.0026,0f000001,0*983cddfa\n\tsystem status\tnormal 2 28.000000 0 0\trobot status\t272.552043\t78.583561\t9.521000\t-0.387614\t1.152152\t-33.294354\t0.249000\t0.089000\n\t\n15:22:48.5\tlog_raw\tgps_raw\t#DUALANTENNAHEADINGA,USB3,0,50.5,FINESTEERING,2107,282186.500,02000000,d426,15824;INSUFFICIENT_OBS,NONE,0.000000000,0.000000000,0.000000000,0.0,0.000000000,0.000000000,\"\",0,0,0,0,00,00,00,00*e63b13e8\n\tsystem status\tnormal 2 28.000000 0 0\trobot status\t272.661232\t78.485942\t9.528800\t-0.361377\t1.190799\t-32.883958\t0.292000\t0.026000\n\t\n15:22:49.0\tlog_raw\tgps_raw\t#INSPVAXA,USB3,0,50.5,FINESTEERING,2107,282187.000,02000000,471d,15824;INS_ALIGNMENT_COMPLETE,INS_RTKFIXED,37.37083651711,126.72391453390,9.5369,22.3000,-0.1989,0.2174,0.0087,-0.266896449,1.151079764,122.361675094,0.6060,0.3885,0.7100,0.1370,0.1076,0.0827,0.1473,0.1517,5.0026,0f000001,0*c07c766a\n\tsystem status\tnormal 2 27.900000 0 0\trobot status\t272.770759\t78.386259\t9.536900\t-0.266896\t1.151080\t-32.361675\t0.322000\t-0.027000\n\t\n15:22:49.5\tlog_raw\tgps_raw\t#DUALANTENNAHEADINGA,USB3,0,50.0,FINESTEERING,2107,282187.500,02000000,d426,15824;INSUFFICIENT_OBS,NONE,0.000000000,0.000000000,0.000000000,0.0,0.000000000,0.000000000,\"\",0,0,0,0,00,00,00,00*f7dadc56\n\tsystem status\tnormal 2 27.900000 0 0\trobot status\t272.879683\t78.288960\t9.544800\t-0.300203\t1.356703\t-31.762016\t0.241000\t0.102000\n\t\n15:22:50.0\tlog_raw\tgps_raw\t#DUALANTENNAHEADINGA,USB3,0,50.0,FINESTEERING,2107,282188.000,02000000,d426,15824;INSUFFICIENT_OBS,NONE,0.000000000,0.000000000,0.000000000,0.0,0.000000000,0.000000000,\"\",0,0,0,0,00,00,00,00*92e72652\n\tsystem status\tnormal 2 27.900000 0 0\trobot status\t272.989156\t78.191427\t9.553900\t-0.243529\t1.456770\t-31.175721\t0.284000\t0.049000\n\t\n15:22:50.5\tlog_raw\tgps_raw\t#DUALANTENNAHEADINGA,USB3,0,53.5,FINESTEERING,2107,282188.500,02000000,d426,15824;INSUFFICIENT_OBS,NONE,0.000000000,0.000000000,0.000000000,0.0,0.000000000,0.000000000,\"\",0,0,0,0,00,00,00,00*10de566f\n\tsystem status\tnormal 2 27.900000 0 0\trobot status\t273.116821\t78.130003\t9.550800\t-0.253253\t1.384149\t-30.556264\t0.163000\t0.228000\n\t\n15:22:51.0\tlog_raw\tgps_raw\t#DUALANTENNAHEADINGA,USB3,0,53.5,FINESTEERING,2107,282189.000,02000000,d426,15824;INSUFFICIENT_OBS,NONE,0.000000000,0.000000000,0.000000000,0.0,0.000000000,0.000000000,\"\",0,0,0,0,00,00,00,00*b94d3568\n\tsystem status\tnormal 2 27.900000 0 0\trobot status\t273.244255\t78.071378\t9.546600\t-0.301830\t1.355616\t-29.874726\t0.377000\t-0.079000\n\t\n15:22:51.5\tlog_raw\tgps_raw\t#DUALANTENNAHEADINGA,USB3,0,51.5,FINESTEERING,2107,282189.500,02000000,d426,15824;INSUFFICIENT_OBS,NONE,0.000000000,0.000000000,0.000000000,0.0,0.000000000,0.000000000,\"\",0,0,0,0,00,00,00,00*706ecbbe\n\tsystem status\tnormal 2 27.900000 0 0\trobot status\t273.362901\t77.999753\t9.547600\t-0.330497\t1.496493\t-29.265586\t0.230000\t0.119000\n\t\n15:22:52.0\tlog_raw\tgps_raw\t#DUALANTENNAHEADINGA,USB3,0,51.5,FINESTEERING,2107,282190.000,02000000,d426,15824;INSUFFICIENT_OBS,NONE,0.000000000,0.000000000,0.000000000,0.0,0.000000000,0.000000000,\"\",0,0,0,0,00,00,00,00*9080aeab\n\tsystem status\tnormal 2 27.900000 0 0\trobot status\t273.483457\t77.925818\t9.549200\t-0.201531\t1.436822\t-28.848585\t0.240000\t0.089000\n\t\n15:22:52.5\tlog_raw\tgps_raw\t#DUALANTENNAHEADINGA,USB3,0,51.5,FINESTEERING,2107,282190.500,02000000,d426,15824;SOL_COMPUTED,NARROW_FLOAT,-1.000000000,135.085830688,-53.305603027,0.0,360.000000000,180.000000000,\"631T\",17,6,6,5,04,00,20,03*0a25629d\n\tsystem status\tnormal 2 28.000000 0 0\trobot status\t273.605331\t77.846855\t9.551100\t-0.000872\t1.141836\t-28.612201\t0.257000\t0.054000\n\t\n15:22:53.0\tlog_raw\tgps_raw\t#DUALANTENNAHEADINGA,USB3,0,51.5,FINESTEERING,2107,282191.000,02000000,d426,15824;SOL_COMPUTED,NARROW_FLOAT,-1.000000000,135.135757446,-54.312408447,0.0,360.000000000,180.000000000,\"631T\",18,6,6,5,04,00,20,03*2fbb2179\n\tsystem status\tnormal 2 28.000000 0 0\trobot status\t273.725524\t77.770330\t9.552900\t-0.136730\t1.098500\t-28.543191\t0.218000\t0.115000\n\t\n15:22:53.5\tlog_raw\tgps_raw\t#DUALANTENNAHEADINGA,USB3,0,51.0,FINESTEERING,2107,282191.500,02000000,d426,15824;SOL_COMPUTED,NARROW_FLOAT,-1.000000000,134.974884033,-69.401855469,0.0,360.000000000,164.567916870,\"631T\",18,7,7,5,04,00,20,03*c918ed4a\n\tsystem status\tnormal 2 28.100000 0 0\trobot status\t273.841224\t77.693882\t9.554400\t-0.238021\t1.170803\t-28.612330\t0.294000\t-0.008000\n\t\n15:22:54.0\tlog_raw\tgps_raw\t#DUALANTENNAHEADINGA,USB3,0,51.0,FINESTEERING,2107,282192.000,02000000,d426,15824;SOL_COMPUTED,NARROW_FLOAT,-1.000000000,134.756271362,-69.514831543,0.0,360.000000000,164.104385376,\"631T\",19,7,7,5,04,00,20,03*4a4dea82\n\tsystem status\tnormal 2 28.100000 0 0\trobot status\t273.954349\t77.616485\t9.556300\t-0.165500\t1.196051\t-28.623420\t0.300000\t-0.021000\n\t\n15:22:54.5\tlog_raw\tgps_raw\t#DUALANTENNAHEADINGA,USB3,0,48.5,FINESTEERING,2107,282192.500,02000000,d426,15824;INSUFFICIENT_OBS,NONE,0.000000000,0.000000000,0.000000000,0.0,0.000000000,0.000000000,\"\",0,0,0,0,00,00,00,00*a4d33cd7\n\tsystem status\tnormal 2 28.100000 0 0\trobot status\t274.069885\t77.537341\t9.557600\t-0.041207\t1.165144\t-28.715617\t0.302000\t-0.020000\n\t\n15:22:55.0\tlog_raw\tgps_raw\t#DUALANTENNAHEADINGA,USB3,0,48.5,FINESTEERING,2107,282193.000,02000000,d426,15824;INSUFFICIENT_OBS,NONE,0.000000000,0.000000000,0.000000000,0.0,0.000000000,0.000000000,\"\",0,0,0,0,00,00,00,00*0d405fd0\n\tsystem status\tnormal 2 28.100000 0 0\trobot status\t274.180328\t77.460560\t9.559600\t-0.000370\t1.224221\t-28.851845\t0.302000\t-0.016000\n\t\n15:22:55.5\tlog_raw\tgps_raw\t#DUALANTENNAHEADINGA,USB3,0,50.5,FINESTEERING,2107,282193.500,02000000,d426,15824;SOL_COMPUTED,NARROW_FLOAT,-1.000000000,151.214721680,75.840576172,0.0,311.274841309,57.009273529,\"631T\",15,8,8,5,04,00,20,03*7af4d743\n\tsystem status\tnormal 2 28.100000 0 0\trobot status\t274.296771\t77.370135\t9.566200\t-0.089150\t1.290239\t-29.092643\t0.306000\t-0.025000\n\t\n15:22:56.0\tlog_raw\tgps_raw\t#DUALANTENNAHEADINGA,USB3,0,50.5,FINESTEERING,2107,282194.000,02000000,d426,15824;SOL_COMPUTED,NARROW_FLOAT,-1.000000000,150.594802856,75.862449646,0.0,315.079772949,56.983615875,\"631T\",15,8,8,5,04,00,20,03*a31139df\n\tsystem status\tnormal 2 28.000000 0 0\trobot status\t274.415573\t77.275380\t9.573700\t-0.145800\t1.170511\t-29.352538\t0.298000\t-0.028000\n\t\n15:22:56.5\tlog_raw\tgps_raw\t#DUALANTENNAHEADINGA,USB3,0,49.5,FINESTEERING,2107,282194.500,02008000,d426,15824;SOL_COMPUTED,NARROW_FLOAT,-1.000000000,75.730995178,-6.270477295,0.0,224.747741699,180.000000000,\"631T\",15,8,8,5,04,00,20,03*aae5cd6a\n\tsystem status\tnormal 2 28.000000 0 0\trobot status\t274.542069\t77.195884\t9.577100\t-0.158234\t1.209867\t-29.626584\t0.299000\t-0.018000\n\t\n15:22:57.0\tlog_raw\tgps_raw\t#DUALANTENNAHEADINGA,USB3,0,49.5,FINESTEERING,2107,282195.000,02008000,d426,15824;SOL_COMPUTED,NARROW_FLOAT,-1.000000000,76.029739380,-7.977203369,0.0,225.982131958,180.000000000,\"631T\",16,8,8,5,04,00,20,03*1aef0704\n\tsystem status\tnormal 2 28.100000 0 0\trobot status\t274.667953\t77.115279\t9.578700\t-0.125238\t1.284653\t-29.931005\t0.294000\t-0.010000\n\t\n15:22:57.5\tlog_raw\tgps_raw\t#DUALANTENNAHEADINGA,USB3,0,50.0,FINESTEERING,2107,282195.500,02008000,d426,15824;INSUFFICIENT_OBS,NONE,0.000000000,0.000000000,0.000000000,0.0,0.000000000,0.000000000,\"\",0,0,0,0,00,00,00,00*3a754bb7\n\tsystem status\tnormal 2 28.100000 0 0\trobot status\t274.790079\t77.032974\t9.580500\t-0.163438\t1.215045\t-30.241931\t0.298000\t-0.032000\n\t\n15:22:58.0\tlog_raw\tgps_raw\t#DUALANTENNAHEADINGA,USB3,0,50.0,FINESTEERING,2107,282196.000,
